vi "Get Kasli Interface.vi"(8 "error in":errorcluster) -> (0 "error out":errorcluster, 3 "Kasli Interface":refnum<class "Kasli.lvclass">)   [LabVIEW 2020, in "Kasli Wrapper 2.0.lvlib"]
uses:
  Kasli Wrapper 2.0.lvlib
  Kasli/Kasli.lvclass
  TALOS/TALOS_PPL.lvlibp/Support VIs/Global Memory.vi
  TALOS/TALOS_PPL.lvlibp
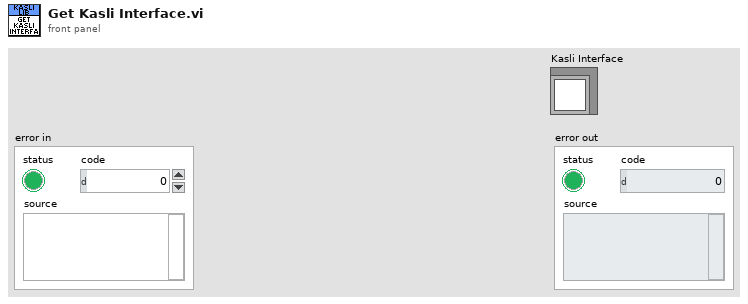
[diagram p1: front panel]
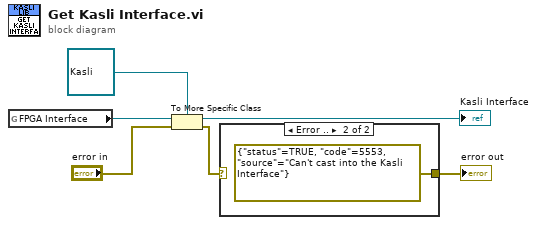
[diagram p0: block diagram]
diagram:
  n1 = global read "Global Memory.vi" "FPGA Interface"() -> (w6:refnum<class "FPGA Interface.lvclass">)
  n2 = To More Specific Class(target class=refnum<class "Kasli.lvclass"> refnum ("Kasli"), reference=w6, error in="error in") -> (specific class reference=→"Kasli Interface":refnum<class "Kasli.lvclass">, error out=w3:errorcluster)
  n3 = case shown="Error .." w3 {
    selector: w3 -> [w7 _]
    tunnel: [w7 errorcluster {"status"=TRUE, "code"=5553, "source"="Can't cast into the Kasli Interface"} ("error IO")] -> w2
    frame No Error {
    }
    frame Error {
    }
  }
  "error out" <- w2
